vi "VI Linearisierung v2.vi"() -> ()   [LabVIEW 2020, in "Linearisierung v2.lvlib"] (continued)
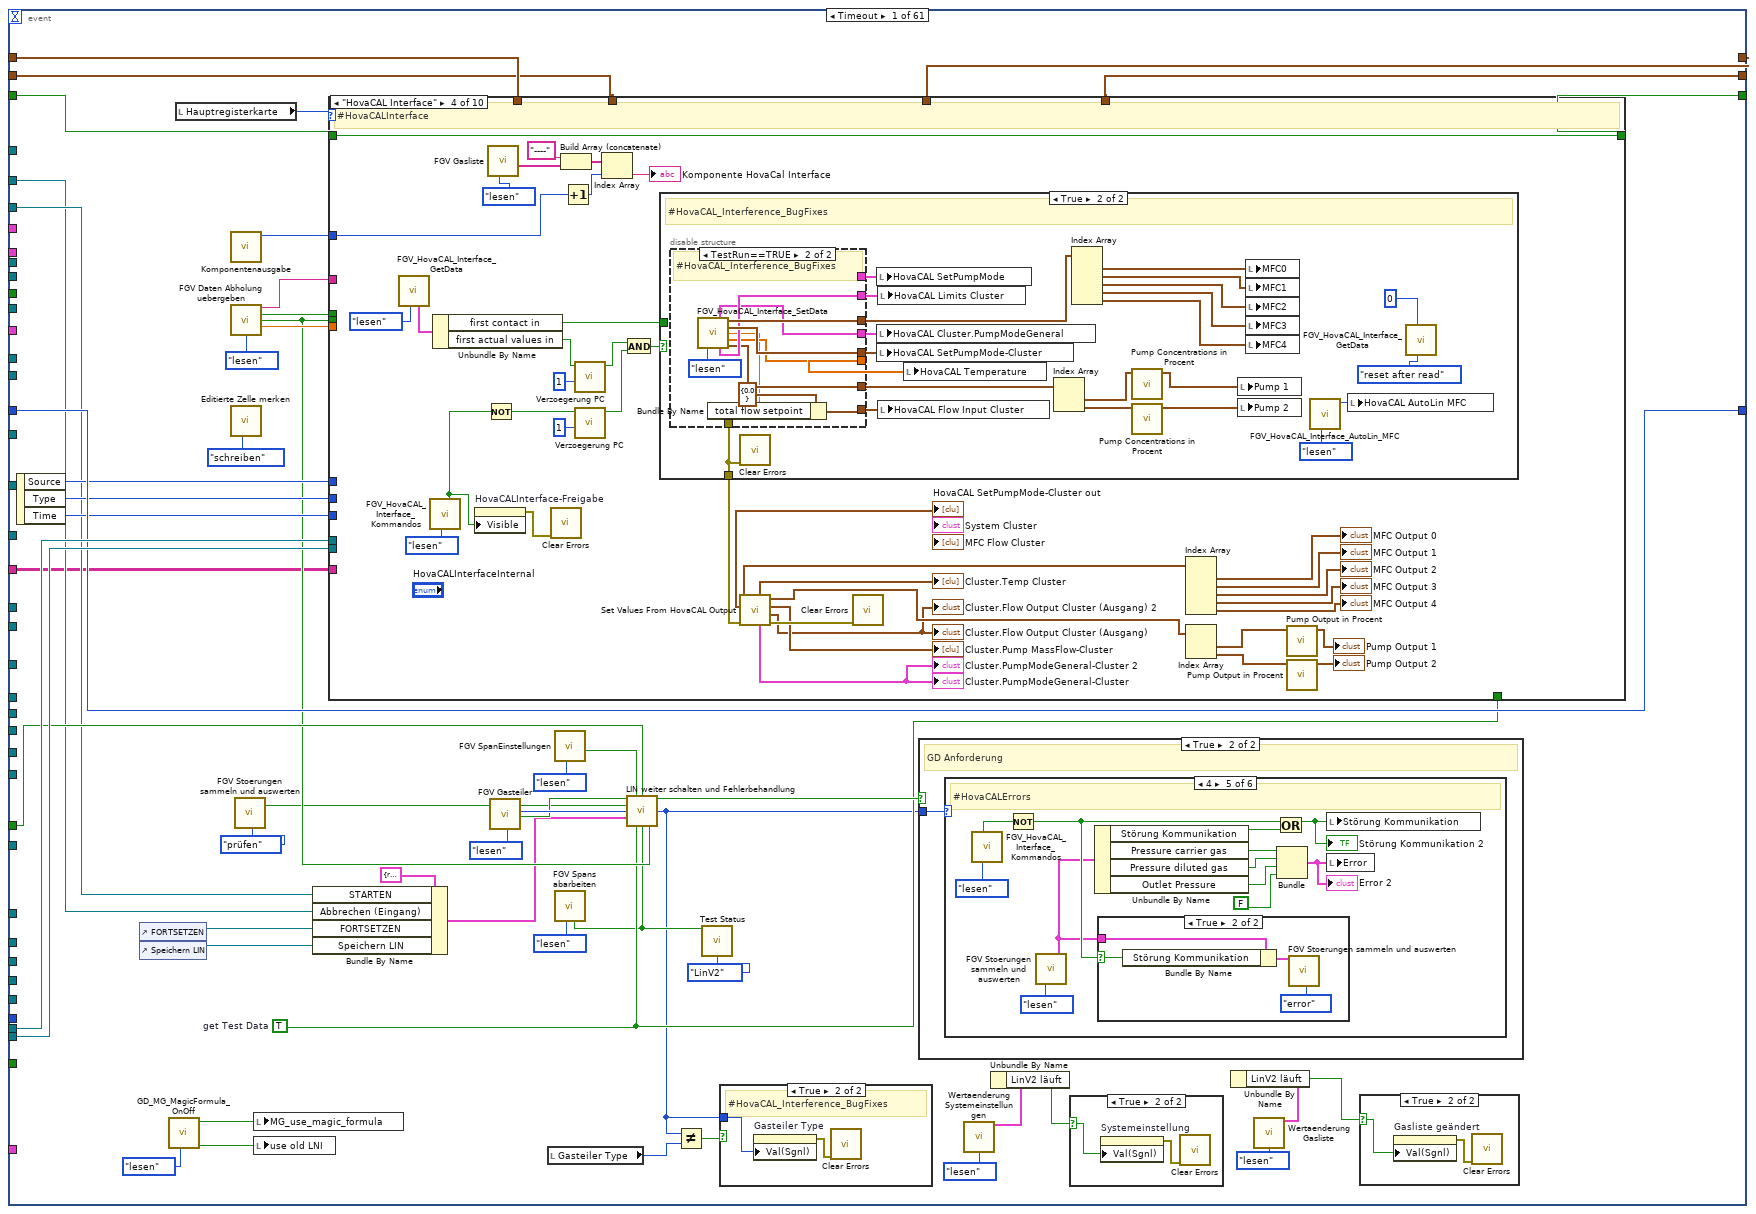
[diagram p2: hidden frame]
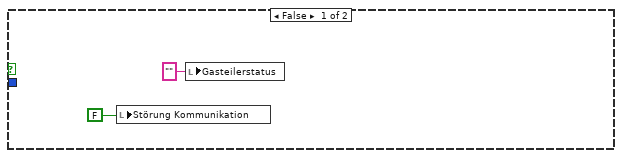
[diagram p6: hidden frame]
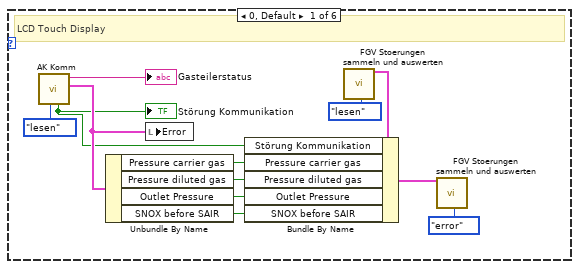
[diagram p7: hidden frame]
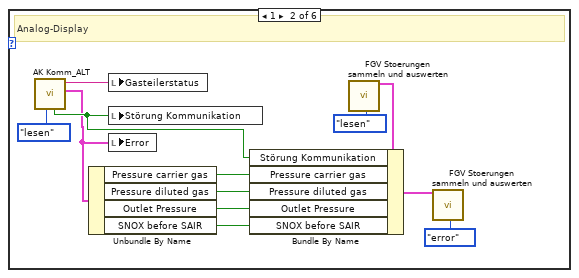
[diagram p8: hidden frame]
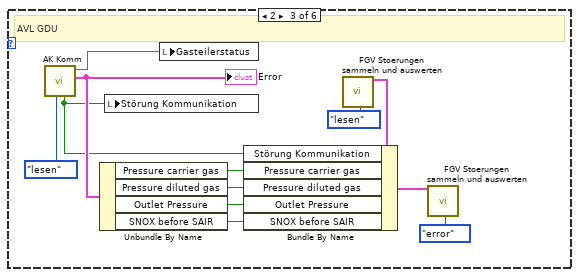
[diagram p9: hidden frame]
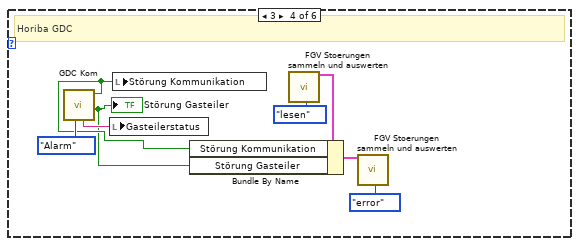
[diagram p10: hidden frame]
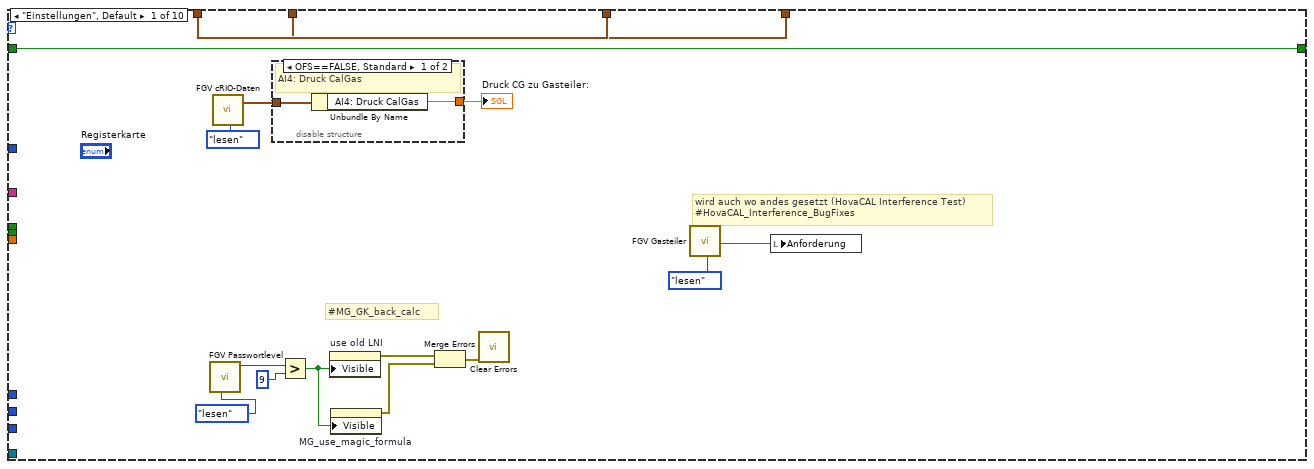
[diagram p13: hidden frame]
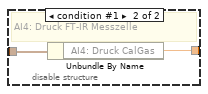
[diagram p14: hidden frame]
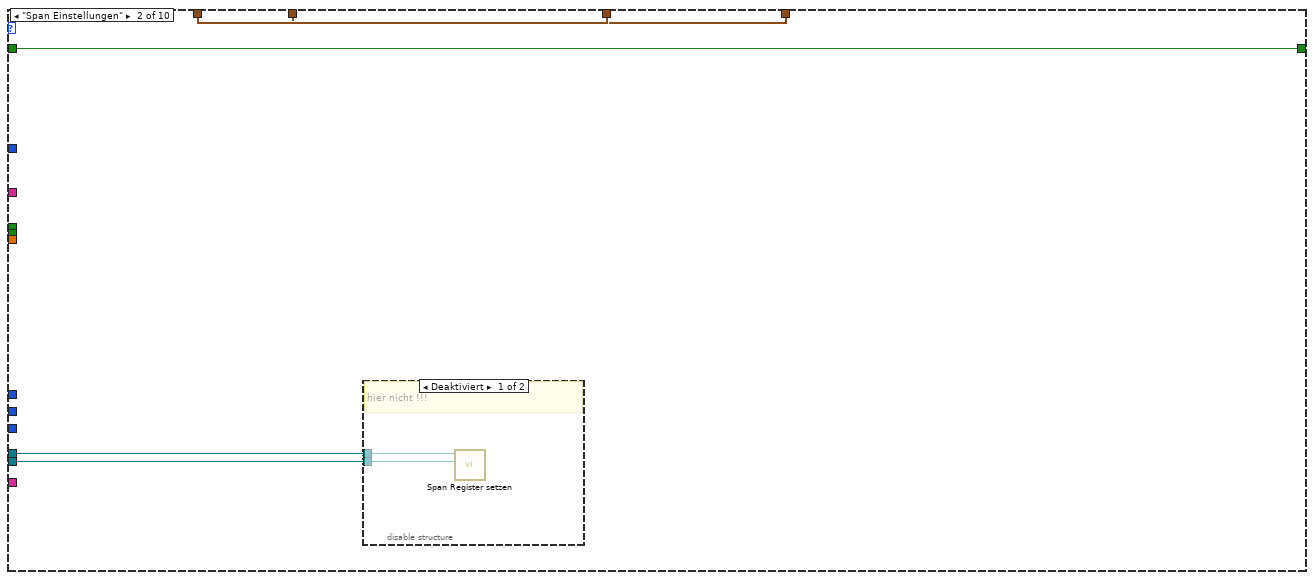
[diagram p15: hidden frame]
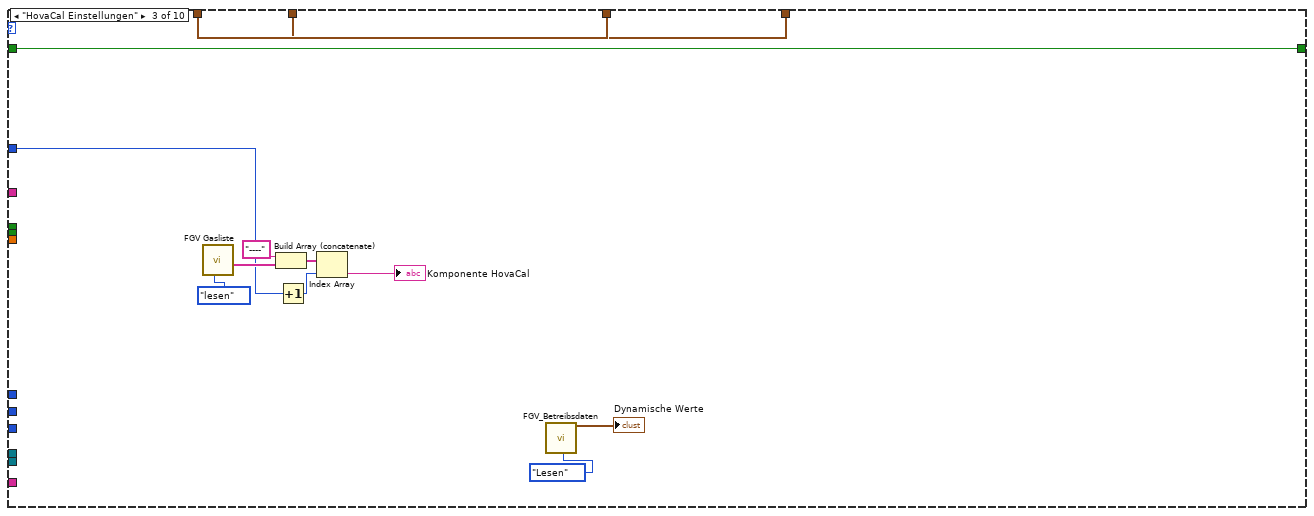
[diagram p17: hidden frame]
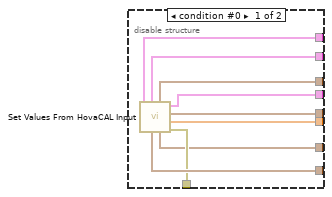
[diagram p19: hidden frame]
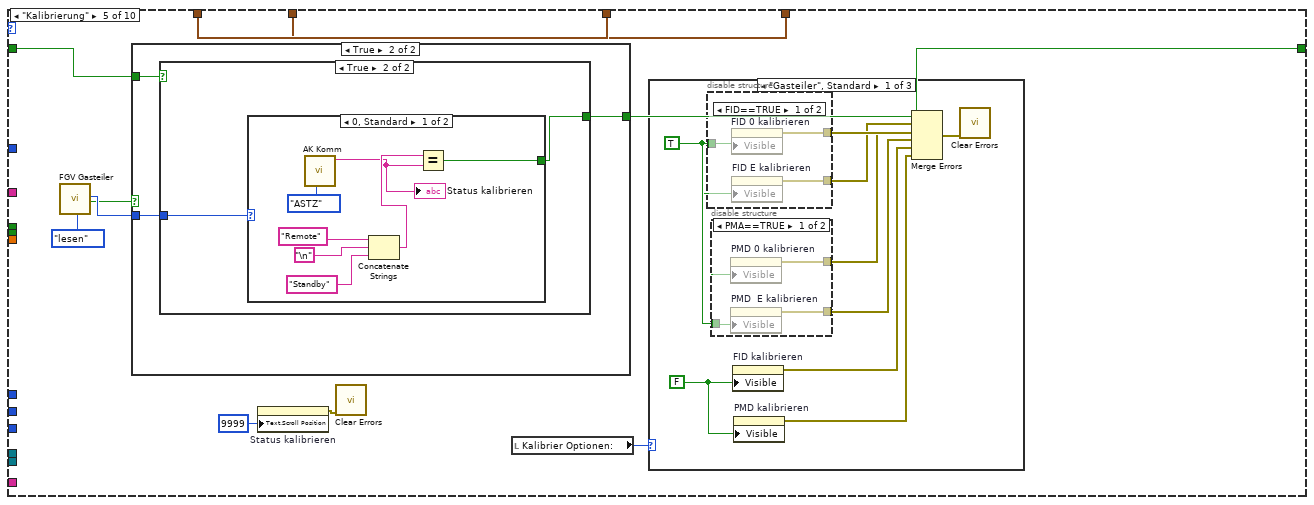
[diagram p20: hidden frame]
                    n2156 = call "FGV_Betreibsdaten.vi"("Enum"=Aktion_FGV_Betriebsdaten."Lesen" ("Aktion")) -> ("Sollwert für Vergleich"=w4010:T64)  [unwired: 11 in, 7 out]
                    n2157 = Bundle By Name(cluster=w4010, "Eingangskonzentration\nKomponente 1"=w4012) -> (w4014:T64)
                    n2158 = call "FGV_Betreibsdaten.vi"("Sollwert schreiben"=w4014, "Enum"=Aktion_FGV_Betriebsdaten."Sollwerte schreiben" ("Aktion")) -> ("Sollwert für Vergleich"=w4011:T64)  [unwired: 10 in, 7 out]
                    n2159 = property on="Daten" class="Cluster (strikt)"("Val(Sgnl)"=w4011) -> (error out=w4013:errorcluster)  [unwired: 2 in, 1 out]
                    n2160 = call <vilib>:"Clear Errors.vi"("error in (no error)"=w4013) -> ()  [unwired: 5 in, 2 out]
                  }
                  frame 2 {
                    n2161 = call "FGV_Betreibsdaten.vi"("Enum"=Aktion_FGV_Betriebsdaten."Lesen" ("Aktion")) -> ("Sollwert für Vergleich"=w4017:T64)  [unwired: 11 in, 7 out]
                    n2162 = Bundle By Name(cluster=w4017, "Eingangskonzentration \nKomponente 2"=w4019) -> (w4021:T64)
                    n2163 = call "FGV_Betreibsdaten.vi"("Sollwert schreiben"=w4021, "Enum"=Aktion_FGV_Betriebsdaten."Sollwerte schreiben" ("Aktion")) -> ("Sollwert für Vergleich"=w4018:T64)  [unwired: 10 in, 7 out]
                    n2164 = property on="Daten" class="Cluster (strikt)"("Val(Sgnl)"=w4018) -> (error out=w4020:errorcluster)  [unwired: 2 in, 1 out]
                    n2165 = call <vilib>:"Clear Errors.vi"("error in (no error)"=w4020) -> ()  [unwired: 5 in, 2 out]
                  }
                }
              }
              frame condition #1 (active) {
                n2166 = call "Expand MFC count 2 max MFC index for Pump index.vi"("AutoLin MFC"=w4025) -> ("Pump"=w4024:bool, "Pump Idx"=w4022:i32)  [unwired: 8 in, 1 out]
                n2167 = call "HovaCAL ppm convert from Component.vi"("Konzentration"=w4028, "Gasnummer"=w4026) -> ("Komponenten Name"=w4023:T48, "Konzentration in ppm"=w4027:dbl)  [unwired: 5 in, 3 out]
                n2168 = case shown="True" w4024 {
                  tunnel: w4027 -> [w4030 _]
                  tunnel: w4025 -> [w4029 _]
                  tunnel: w4023 -> [_ w4032]
                  tunnel: w4022 -> [_ w4031]
                  frame False {
                    # "gas"
                    n2169 = call "HovaCAL_Interface_SetComponentConcentration.vi"("AutoLin MFV Index"=w4029, "Konzentration"=w4030) -> ()  [unwired: 7 in, 3 out]
                  }
                  frame True {
                    # "water/reagent"
                    n2170 = call "HovaCAL_Interface_SetPumpParameter.vi"("Pump Idx"=w4031, "Komponent Name"=w4032) -> ()  [unwired: 9 in, 1 out]
                  }
                }
              }
            }
          }
        }
        n2171 = local write "LIN Polynomkoeffizienten"(w3935) -> ()
        n2172 = Index Array(array=w3899, index=w3900) -> (element=w3898:refnum<vi>)
        n2173 = local write "EPA Ausgabetabelle"(w3939) -> ()
        n2174 = local write "LIN Ausgabetabelle"(w3936) -> ()
        n2175 = local write "EPA Auswertung"(w3937) -> ()
        n2176 = local write "XY-Graph EPA"(w3938) -> ()
        n2177 = property class="Tbl (strikt)"(reference=w3898, "Value"=w3897) -> (error out=w3896:errorcluster)  [unwired: 1 in, 1 out]
        n2178 = local write "Aktiv"(w3940) -> ()
        n2179 = call <vilib>:"Clear Errors.vi"("error in (no error)"=w3896) -> ()  [unwired: 5 in, 2 out]
      }
      event Value Change {
        # "Stufenaufteilung immer nur nach 1. Komponente ?!\nFormel daher auch ...\naus Gaxsliste oder aus \"vereinzeln\" ?"
        # "-> Bearbeiter -> Gasnummer generieren"
        n2180 = event-data() -> ()  [unwired: 1 in, 6 out]
        n2181 = Build Array("Span 1", "Span 2", "Span 3", "Span 4", "Span 5", "Span 6", "Span 7", "Span 8", "Span 9", "Span 10") -> (w4064:T19[])
        n2182 = call "FGV SpanEinstellungen.vi"("Aktion"=Aktion_FGV_SpanEinstellungen."lesen") -> ("SpanInletClusterArray out"=w4062:T19[])  [unwired: 6 in, 4 out]
        n2183 = for {
          tunnel: w4065 -> [w4094] mode=indexing
          tunnel: w4064 -> [w4088] mode=indexing
          tunnel: w4062 -> [w4093] mode=indexing
          tunnel: [w4087] -> w4049 mode=indexing
          n2184 = call "FGV SPAN Verriegelung.vi"("aktion"=Aktion_FGV_SPAN_Verriegelung."lesen") -> ("locked"=w4081:bool)  [unwired: 8 in, 2 out]
          n2185 = Unbundle By Name(w4088) -> ("Konfig Gasflasche"=w4091:T20, "Komponenten"=w4085:T23, "Gasflasche"=w4089:T22)
          n2186 = Unbundle By Name(w4093) -> ("Komponenten"=w4086:T23, "Gasflasche"=w4092:T22)
          n2187 = case shown="False" w4081 {
            tunnel: w4094 -> [w4096 _]
            tunnel: w4091 -> [w4095 _]
            frame False {
              n2188 = call "Konfig Gasflasche aktiv.vi"("Konfig Gasflasche"=w4095, "Referenz Gasflasche"=w4096) -> ("error out"=w4097:errorcluster)  [unwired: 9 in]
              n2189 = call <vilib>:"Clear Errors.vi"("error in (no error)"=w4097) -> ()  [unwired: 5 in, 2 out]
            }
            frame True {
            }
          }
          n2190 = Not Equal?(x=w4089, y=w4092) -> (x != y?=w4090:bool)
          n2191 = Not Equal?(x=w4085, y=w4086) -> (x != y?=w4083:bool)
          n2192 = And(x=w4091, y=w4090) -> (x .and. y?=w4082:T20)
          n2193 = case shown="False" w4083 {
            tunnel: w4089 -> [w4101 _]
            tunnel: w4088 -> [w4100 w4109]
            tunnel: [w4099 w4108] -> w4087
            tunnel: w4086 -> [_ w4110]
            tunnel: w4085 -> [_ w4107]
            tunnel: w4082 -> [w4098 _]
            frame False {
              n2194 = case shown="True" w4098 {
                tunnel: w4101 -> [_ w4105]
                tunnel: w4100 -> [w4102 w4104]
                tunnel: [w4102 w4103] -> w4099
                frame False {
                }
                frame True {
                  n2195 = call "Spaneinstellung befuellen.vi"("Gasflasche"=w4105, "Span 1"=w4104) -> ("Span 1"=w4103:T19)  [unwired: 7 in, 2 out]
                }
              }
            }
            frame True {
              n2196 = call "Komponenten Formeln Finden.vi"("Komponenten Alt"=w4110, "Komponenten (Eingang)"=w4107) -> ("Komponenten (Ausgang)"=w4106:T23)  [unwired: 9 in]
              n2197 = Bundle By Name(cluster=w4109, "Komponenten"=w4106) -> (w4108:T19)
            }
          }
        }
        n2198 = call "get Summenformeln and update.vi"("SpanInletClusterArray in"=w4049) -> ("error out"=w4047:errorcluster, "Summenformeln 1.Komponente"=w4046:T12[], "SpanInletClusterArray out"=w4048:T19[])  [unwired: 7 in, 1 out]
        n2199 = Index Array(array=w4046) -> (element #1=w4045:T12, element #2=w4044:T12, element #3=w4043:T12, element #4=w4042:T12, element #5=w4041:T12, element #6=w4040:T12, element #7=w4039:T12, element #8=w4038:T12, element #9=w4037:T12, element #10=w4036:T12)  [unwired: 10 in]
        n2200 = call "FGV SpanEinstellungen.vi"("Aktion"=Aktion_FGV_SpanEinstellungen."schreiben", "error in (no error)"=w4047, "SpanInletClusterArray in"=w4048) -> ("error out"=w4066:errorcluster, "SpanInletClusterArray out"=w4051:T19[])  [unwired: 4 in, 3 out]
        n2201 = local write "PrüfgasName"(w4045) -> ()
        n2202 = local write "PrüfgasName 2"(w4044) -> ()
        n2203 = local write "PrüfgasName 3"(w4043) -> ()
        n2204 = local write "PrüfgasName 4"(w4042) -> ()
        n2205 = local write "PrüfgasName 5"(w4041) -> ()
        n2206 = local write "PrüfgasName 6"(w4040) -> ()
        n2207 = local write "PrüfgasName 7"(w4039) -> ()
        n2208 = local write "PrüfgasName 8"(w4038) -> ()
        n2209 = local write "PrüfgasName 9"(w4037) -> ()
        n2210 = local write "PrüfgasName 10"(w4036) -> ()
        n2211 = call "FGV SpanEinstellungen.vi"("Aktion"=Aktion_FGV_SpanEinstellungen."speichern", "error in (no error)"=w4066, "SpanInletClusterArray in"=w4051) -> ("automatisch out"=w4035:T20, "SpanInletClusterArray out"=w4050:T19[])  [unwired: 4 in, 3 out]
        n2212 = Index Array(array=w4050) -> (element #1=w4061:T19, element #2=w4060:T19, element #3=w4059:T19, element #4=w4058:T19, element #5=w4057:T19, element #6=w4056:T19, element #7=w4055:T19, element #8=w4054:T19, element #9=w4053:T19, element #10=w4052:T19)  [unwired: 10 in]
        n2213 = local write "Span 1"(w4061) -> ()
        n2214 = local write "Span 2"(w4060) -> ()
        n2215 = local write "Span 3"(w4059) -> ()
        n2216 = local write "Span 4"(w4058) -> ()
        n2217 = local write "Span 5"(w4057) -> ()
        n2218 = local write "Span 6"(w4056) -> ()
        n2219 = local write "Span 7"(w4055) -> ()
        n2220 = local write "Span 8"(w4054) -> ()
        n2221 = local write "Span 9"(w4053) -> ()
        n2222 = local write "Span 10"(w4052) -> ()
        n2223 = call "Bearbeiter_triggern.vi"("automatisch out"=w4035, "Bearbeiter (Eingang)"=w4034) -> ()  [unwired: 10 in]
      }
      event Value Change {
        n2224 = event-data() -> ()  [unwired: 1 in, 1 out]
        n2225 = vi-ref "Gasteiler Korrektur.vi"() -> (w4113:refnum<vi>)
        n2226 = call "VI Pop Up.vi"("VI Referenz"=w4113) -> ()  [unwired: 10 in, 1 out]
      }
      event Value Change {
        n2227 = event-data() -> ()  [unwired: 1 in, 1 out]
        n2228 = case shown="True" "Istwerte löschen" {
          tunnel: [_ w4136] -> w4133
          frame False {
          }
          frame True {
            n2229 = call "Lin Daten aufarbeiten.vi"("Aktionen"=Aktion_Lin_Daten_aufarbeiten."Istwerte löschen") -> ("error out"=w4136:errorcluster)  [unwired: 16 in, 10 out]
          }
        }
        n2230 = case shown="True" "Alles löschen" {
          tunnel: [_ w4138] -> w4132
          frame False {
          }
          frame True {
            n2231 = call "Lin Daten aufarbeiten.vi"("Aktionen"=Aktion_Lin_Daten_aufarbeiten."Tabelle löschen") -> ("error out"=w4138:errorcluster)  [unwired: 16 in, 10 out]
          }
        }
        n2232 = Merge Errors(w4133, w4132) -> (w4124:errorcluster)
        n2233 = call "Komponentenausgabe.vi"() -> ("Gaskomponente"=w4119:T7)  [unwired: 8 in, 3 out]
        n2234 = call "Lin Daten aufarbeiten.vi"("Index (Seite)"=w4119, "error in (no error)"=w4124, "Aktionen"=Aktion_Lin_Daten_aufarbeiten."EPA auswerten") -> ("Index (Seite) out"=w4118:i32, "error out"=w4123:errorcluster)  [unwired: 14 in, 9 out]
        n2235 = call "Lin Daten aufarbeiten.vi"("Index (Seite)"=w4118, "error in (no error)"=w4123, "Polynom-Ordnung"=Auswahl_Polynom_Ordnung."actual", "Aktionen"=Aktion_Lin_Daten_aufarbeiten."Lin auswerten") -> ("Index (Seite) out"=w4117:i32, "error out"=w4122:errorcluster)  [unwired: 13 in, 9 out]
        n2236 = call "Lin Daten aufarbeiten.vi"("Index (Seite)"=w4117, "error in (no error)"=w4122, "Aktionen"=Aktion_Lin_Daten_aufarbeiten."lesen") -> ("Eingabetabelle"=w4130:T54, "error out"=w4131:errorcluster)  [unwired: 14 in, 9 out]
        n2237 = call "AusgabeTabelle zusammenbauen.vi"("error in (no error)"=w4131, "Eingabetabelle"=w4130) -> ("Eingabetabelle behandelt"=w4127:string[][], "Ausgabetabelle"=w4128:T53)  [unwired: 7 in, 1 out]
        n2238 = local write "Ausgabetabelle"(w4128) -> ()
        n2239 = local write "Eingabetabelle"(w4127) -> ()
      }
      event Value Change {
        n2240 = event-data() -> ()  [unwired: 1 in, 1 out]
        n2241 = local read "Gasteiler Type"() -> (w4144:T15)
        n2242 = call "FGV Gasteiler.vi"("Serielle Parameter"="Serielle Parameter", "Aktionen"=Aktionen_FGV_Gasteiler_Daten."Seriellen Param.") -> ("Serielle Parameter"=w4148:T129)  [unwired: 10 in, 7 out]
        n2243 = call "FGV Gasteiler.vi"("Serielle Parameter"=w4148, "Aktionen"=Aktionen_FGV_Gasteiler_Daten."speichern") -> ("Serielle Parameter"=w4141:T129)  [unwired: 10 in, 7 out]
        n2244 = case shown="4" w4144 {
          tunnel: w4141 -> [_ w4150]
          frame 0, Default {
          }
          frame 4 {
            # "#HovaCALInterface"
            n2245 = Unbundle By Name(w4150) -> ("VISA resource name"=w4149:refnum<visa-resource-name>)
            n2246 = call "FGV Gasteiler.vi"("Aktionen"=Aktionen_FGV_Gasteiler_Daten."lesen") -> ("Anforderung"=w4151:bool)  [unwired: 11 in, 7 out]
            n2247 = case shown="True" w4151 {
              tunnel: w4149 -> [w4153 w4159]
              frame False {
                n2248 = disable-structure shown="HovaCALInterface==TRUE, Standard" {
                  disable-tunnel: w4153 -> [w4154 _]
                  frame condition #0 {
                    n2249 = call "FGV_Kommunikation.vi"("Aktion"=Aktion_FGV_Kom."Com ändern", "VISA"=w4154) -> ("error out"=w4155:errorcluster)  [unwired: 5 in, 4 out]
                    n2250 = call <vilib>:"Clear Errors.vi"("error in (no error)"=w4155) -> ()  [unwired: 5 in, 2 out]
                  }
                  frame condition #1 (active) {
                    n2251 = call "FGV_HovaCAL_Interface_Kommandos.vi"("Aktion"=Aktion_FGV_HovaCAL_Interface_Kommandos."on top", "Kommando in"=Aktion_FGV_HovaCAL_Interface_Kommunikation."Com ändern" ("Kommando")) -> ()  [unwired: 3 in, 6 out]
                  }
                }
              }
              frame True {
                n2252 = stacked-sequence {
                  tunnel: w4159 -> [w4160 _ _]
                  frame #0 {
                    n2253 = disable-structure shown="HovaCALInterface==TRUE, Standard" {
                      disable-tunnel: w4160 -> [w4161 _]
                      frame condition #0 {
                        n2254 = call "FGV_Kommunikation.vi"("Aktion"=Aktion_FGV_Kom."Beenden") -> ("error out"=w4165:errorcluster)  [unwired: 6 in, 4 out]
                        n2255 = call "FGV_Kommunikation.vi"("error in"=w4165, "Aktion"=Aktion_FGV_Kom."Com ändern", "VISA"=w4161) -> ("error out"=w4163:errorcluster)  [unwired: 4 in, 4 out]
                        n2256 = call "FGV_Kommunikation.vi"("error in"=w4163, "Aktion"=Aktion_FGV_Kom."Initialisieren") -> ("error out"=w4162:errorcluster)  [unwired: 5 in, 4 out]
                        n2257 = call <vilib>:"Clear Errors.vi"("error in (no error)"=w4162) -> ()  [unwired: 5 in, 2 out]
                      }
                      frame condition #1 (active) {
                        n2258 = call "FGV_HovaCAL_Interface_Kommandos.vi"("Aktion"=Aktion_FGV_HovaCAL_Interface_Kommandos."on top", "Kommando in"=Aktion_FGV_HovaCAL_Interface_Kommunikation."Com ändern" ("Kommando")) -> ("error out"=w4168:errorcluster)  [unwired: 3 in, 5 out]
                        n2259 = disable-structure shown="Deaktiviert" {
                          disable-tunnel: w4168 -> [w4171 _]
                          frame Disabled {
                            n2260 = call "FGV_HovaCAL_Interface_Kommandos.vi"("Aktion"=Aktion_FGV_HovaCAL_Interface_Kommandos."on top", "error in"=w4171, "Kommando in"=Aktion_FGV_HovaCAL_Interface_Kommunikation."Beenden" ("Kommando")) -> ()  [unwired: 2 in, 6 out]
                          }
                          frame Enabled {
                          }
                        }
                      }
                    }
                  }
                  frame #1 {
                    n2261 = disable-structure shown="HovaCALInterface==TRUE, Standard" {
                      frame condition #0 {
                        n2262 = Wait (ms)(milliseconds to wait=u32 2000 ("Zu wartende ms")) -> ()  [unwired: 1 out]
                      }
                      frame condition #1 (active) {
                      }
                    }
                  }
                  frame #2 {
                    n2263 = disable-structure shown="HovaCALInterface==FALSE" {
                      frame condition #0 {
                        n2264 = call "FGV_Kommunikation.vi"("Aktion"=Aktion_FGV_Kom."Gase init") -> ("error out"=w4178:errorcluster, "Gase"=w4176:cluster{string, i32}[][])  [unwired: 6 in, 3 out]
                        n2265 = call "FGV_Betreibsdaten.vi"("Strings und Werte"=w4176, "error in (no error)"=w4178, "Enum"=Aktion_FGV_Betriebsdaten."Gase aendern") -> ("error out"=w4177:errorcluster)  [unwired: 9 in, 7 out]
                        n2266 = call <vilib>:"Clear Errors.vi"("error in (no error)"=w4177) -> ()  [unwired: 5 in, 2 out]
                      }
                      frame condition #1 (active) {
                      }
                    }
                  }
                }
              }
            }
          }
        }
      }
      event "Gasteiler Span Eingänge": Value Change {
        # "#Option10xSpanAuto"
        n2267 = event-data() -> ()  [unwired: 1 in, 1 out]
        n2268 = call "Lin Daten aufarbeiten.vi"("Aktionen"=Aktion_Lin_Daten_aufarbeiten."lesen") -> ("Lin-Polynom"=w4235:T119)  [unwired: 16 in, 10 out]
        n2269 = Bundle By Name(cluster=w4235, "Kalibrator (Gasteiler)"="Gasteiler") -> (w4232:T119)
        n2270 = case shown="4" "Gasteiler Type" {
          selector: "Gasteiler Type" -> [w4285 _ _ _]
          tunnel: "Gasteiler Stufen" -> [w4291 w4300 w4309 _]
          tunnel: [w4291 w4300 w4309 w4322] -> w4228
          tunnel: [FALSE w4299 w4305 w4313] -> w4194
          tunnel: [w4288 w4299 w4307 w4313] -> w4209
          tunnel: [w4288 w4299 w4307 w4313] -> w4208
          tunnel: [w4289 w4298 w4308 TRUE] -> w4207
          tunnel: [w4288 w4299 w4307 w4313] -> w4206
          tunnel: [w4288 w4298 w4307 w4313] -> w4205
          tunnel: [w4288 w4298 w4307 w4313] -> w4204
          tunnel: [w4288 w4299 w4307 w4313] -> w4203
          tunnel: [w4288 w4299 w4307 w4313] -> w4202
          tunnel: [w4288 w4299 w4306 w4313] -> w4201
          tunnel: [w4288 w4299 w4306 w4313] -> w4200
          tunnel: [w4288 w4299 w4306 w4313] -> w4199
          tunnel: [w4288 w4299 w4306 w4313] -> w4198
          tunnel: [w4288 w4299 w4306 w4313] -> w4197
          tunnel: [w4288 w4299 w4305 w4313] -> w4196
          tunnel: [w4288 w4298 w4307 w4313] -> w4195
          tunnel: [FALSE _ TRUE _] -> w4193
          tunnel: w4192 -> [w4277 w4295 w4301 _]
          tunnel: [w4277 w4295 w4301 w4311] -> w4188
          tunnel: w4191 -> [w4286 w4294 w4303 _]
          tunnel: [w4286 w4294 w4303 w4313] -> w4190
          tunnel: "Gasteiler Span Eingänge" -> [w4282 _ w4302 _]
          tunnel: [w4281 0 ("y") w4302 0 ("y")] -> w4186
          tunnel: [w4278 T66."Disabled and Grayed Out" ("Deaktiviert") w4301 w4311] -> w4181
          frame 0..2, Default {
            w4284 = T15 0 items=["LNI", "Analog-Display", "AVL GDU", "Horiba GDC", "HovaCal", "Horiba SGD 710C"] ("x")
            w4288 = TRUE
            # "LCD-Touch Display - Analog Display - AVL GDU"
            n2271 = Equal?(x=w4284, y=w4285) -> (x = y?=w4283:bool)
            n2272 = Select(t=w4277, s=w4283, f=T66."Disabled and Grayed Out" ("Deaktiviert")) -> (s? t:f=w4278:T66)
            n2273 = Not(x=w4288) -> (.not. x?=w4289:bool)
            n2274 = Select(t=w4282, s=w4283, f=u16 0) -> (s? t:f=w4281:u16)
          }
          frame 3 {
            w4296 = FALSE ("Boolesch")
            w4299 = TRUE
            w4298 = FALSE
            # "Horiba GDC"
            n2275 = Boolean To (0,1)(Boolean=w4296) -> (0, 1=w4297:i16)
            n2276 = local write "TCP Verbindung aktiv"(w4296) -> ()
            n2277 = local write "Registerkarte"(w4297) -> ()
          }
          frame 4 {
            w4305 = FALSE
            w4307 = TRUE
            # "Hovacal"
            n2278 = disable-structure shown="HovaCALInterface==TRUE, Standard" {
              disable-tunnel: [TRUE _] -> w4306
              frame condition #0 (active) {
              }
              frame condition #1 {
              }
            }
            n2279 = Not(x=w4307) -> (.not. x?=w4308:bool)
          }
          frame 5 {
            w4311 = T66."Disabled and Grayed Out" ("Deaktiviert")
            w4313 = FALSE
            w4322 = T16 10 items=["10"=10, "16"=16, "32"=32, "64"=64, "128"=128, "256"=256, "500"=500] ("Gasteiler Stufen")
            # "Horiba SGD 710C (manuell)"
            n2280 = local write "Gasteiler Stufen"(w4322) -> ()
            n2281 = call "FGV SpanEinstellungen.vi"("Aktion"=Aktion_FGV_SpanEinstellungen."lesen") -> ("SpanInletClusterArray out"=w4319:T19[])  [unwired: 6 in, 4 out]
            n2282 = To Single Precision Float(number=w4322) -> (single precision float=w4318:sgl)
            n2283 = for {
              tunnel: w4319 -> [w4325] mode=indexing
              tunnel: w4318 -> [w4324]
              tunnel: [w4323] -> w4316 mode=indexing
              n2284 = Bundle By Name(cluster=w4325, "Anzahl Stufen"=w4324) -> (w4323:T19)
            }
            n2285 = call "FGV SpanEinstellungen.vi"("Aktion"=Aktion_FGV_SpanEinstellungen."schreiben", "SpanInletClusterArray in"=w4316) -> ("error out"=w4314:errorcluster)  [unwired: 5 in, 4 out]
            n2286 = call "FGV SpanEinstellungen.vi"("Aktion"=Aktion_FGV_SpanEinstellungen."speichern", "error in (no error)"=w4314) -> ()  [unwired: 5 in, 5 out]
          }
        }
        n2287 = call "Lin Daten aufarbeiten.vi"("Lin-Polynom"=w4232, "Aktionen"=Aktion_Lin_Daten_aufarbeiten."Protkolldaten") -> ()  [unwired: 15 in, 11 out]
        n2288 = case shown="False" w4193 {
          frame True {
            n2289 = control-ref of="Hauptregisterkarte"() -> (w4246:refnum<vi>)
            n2290 = property class="RKElem (strikt)"(reference=w4246) -> (error out=w4249:errorcluster, "Pages"=w4247:refnum<vi>[])  [unwired: 1 in, 1 out]
            n2291 = To Word Integer(number=T8."HovaCal Einstellungen" ("Hauptregisterkarte")) -> (16bit integer=w4245:i16)
            n2292 = Index Array(array=w4247, index #1=w4245, index #2=T8."HovaCAL Interface" ("Hauptregisterkarte")) -> (element #1=w4248:refnum<vi>, element #2=w4250:refnum<vi>)
            n2293 = disable-structure shown="HovaCALInterface==TRUE, Standard" {
              disable-tunnel: w4248 -> [w4257 w4264]
              disable-tunnel: w4249 -> [w4252 w4259]
              disable-tunnel: w4250 -> [w4253 w4260]
              frame condition #0 (active) {
                n2294 = property class="Seite"(reference=w4257, error in=w4252, "PageVis"=FALSE ("Seite sichtbar")) -> (error out=w4255:errorcluster)  [unwired: 1 out]
                n2295 = property class="Seite"(reference=w4253, error in=w4252, "PageVis"=TRUE ("Seite sichtbar")) -> (error out=w4254:errorcluster)  [unwired: 1 out]
                n2296 = call <vilib>:"Clear Errors.vi"("error in (no error)"=w4255) -> ()  [unwired: 5 in, 2 out]
                n2297 = call <vilib>:"Clear Errors.vi"("error in (no error)"=w4254) -> ()  [unwired: 5 in, 2 out]
              }
              frame condition #1 {
                n2298 = property class="Seite"(reference=w4264, error in=w4259, "PageVis"=TRUE ("Seite sichtbar")) -> (error out=w4262:errorcluster)  [unwired: 1 out]
                n2299 = property class="Seite"(reference=w4260, error in=w4259, "PageVis"=FALSE ("Seite sichtbar")) -> (error out=w4261:errorcluster)  [unwired: 1 out]
                n2300 = call <vilib>:"Clear Errors.vi"("error in (no error)"=w4262) -> ()  [unwired: 5 in, 2 out]
                n2301 = call <vilib>:"Clear Errors.vi"("error in (no error)"=w4261) -> ()  [unwired: 5 in, 2 out]
              }
            }
          }
          frame False {
            n2302 = control-ref of="Hauptregisterkarte"() -> (w4272:refnum<vi>)
            n2303 = property class="RKElem (strikt)"(reference=w4272) -> (error out=w4275:errorcluster, "Pages"=w4273:refnum<vi>[])  [unwired: 1 in, 1 out]
            n2304 = To Word Integer(number=T8."HovaCal Einstellungen" ("Hauptregisterkarte")) -> (16bit integer=w4271:i16)
            n2305 = Index Array(array=w4273, index #1=w4271, index #2=T8."HovaCAL Interface" ("Hauptregisterkarte")) -> (element #1=w4274:refnum<vi>, element #2=w4276:refnum<vi>)
            n2306 = property class="Seite"(reference=w4274, error in=w4275, "PageVis"=FALSE ("Seite sichtbar")) -> (error out=w4269:errorcluster)  [unwired: 1 out]
            n2307 = property class="Seite"(reference=w4276, error in=w4275, "PageVis"=FALSE ("Seite sichtbar")) -> (error out=w4268:errorcluster)  [unwired: 1 out]
            n2308 = call <vilib>:"Clear Errors.vi"("error in (no error)"=w4269) -> ()  [unwired: 5 in, 2 out]
            n2309 = call <vilib>:"Clear Errors.vi"("error in (no error)"=w4268) -> ()  [unwired: 5 in, 2 out]
          }
        }
        n2310 = call "FGV Gasteiler.vi"("Aktionen"=Aktionen_FGV_Gasteiler_Daten."lesen") -> ("Gasteiler Daten"=w4241:T118)  [unwired: 11 in, 7 out]
        n2311 = Bundle By Name(cluster=w4241, "Gasteiler"="Gasteiler", "Gasteiler Stufen"=w4228, "Gasteiler Type"="Gasteiler Type", "Gasteiler Span Eingänge"=w4186) -> (w4242:T118)
        n2312 = property on="Störung Gasteiler" class="Bool. (strikt)"("Visible"=w4196) -> (error out=w4225:errorcluster)  [unwired: 2 in, 1 out]
        n2313 = property on="Horiba GDC" class="Bool."("Visible"=w4194) -> (error out=w4226:errorcluster)  [unwired: 2 in, 1 out]
        n2314 = property on="STARTEN" class="Bool. (strikt)"("Visible"=w4208) -> (error out=w4210:errorcluster)  [unwired: 2 in, 1 out]
        n2315 = property on="parity" class="Ring (strikt)"("Visible"=w4199) -> (error out=w4220:errorcluster)  [unwired: 2 in, 1 out]
        n2316 = property on="stop bits" class="Ring (strikt)"("Visible"=w4200) -> (error out=w4221:errorcluster)  [unwired: 2 in, 1 out]
        n2317 = property on="Baud Rate" class="Ring (strikt)"("Visible"=w4197) -> (error out=w4222:errorcluster)  [unwired: 2 in, 1 out]
        n2318 = property on="flow control" class="Ring (strikt)"("Visible"=w4201) -> (error out=w4223:errorcluster)  [unwired: 2 in, 1 out]
        n2319 = property on="data bits" class="Ring (strikt)"("Visible"=w4198) -> (error out=w4224:errorcluster)  [unwired: 2 in, 1 out]
        n2320 = property on="Gasteilerkorrektur" class="Bool."("Visible"=w4207) -> (error out=w4212:errorcluster)  [unwired: 2 in, 1 out]
        n2321 = property on="Registerkarte" class="RKElem (strikt)"("Visible"=w4202) -> (error out=w4218:errorcluster)  [unwired: 2 in, 1 out]
        n2322 = property on="Error" class="Cluster (strikt)"("Visible"=w4195) -> (error out=w4217:errorcluster)  [unwired: 2 in, 1 out]
        n2323 = property on="Störung Kommunikation" class="Bool. (strikt)"("Visible"=w4203) -> (error out=w4216:errorcluster)  [unwired: 2 in, 1 out]
        n2324 = property on="TCP Verbindung aktiv" class="Bool. (strikt)"("Visible"=w4204) -> (error out=w4215:errorcluster)  [unwired: 2 in, 1 out]
        n2325 = property on="Error" class="Cluster (strikt)"("Visible"=w4205) -> (error out=w4214:errorcluster)  [unwired: 2 in, 1 out]
        n2326 = property on="automatisch" class="Bool. (strikt)"("Val(Sgnl)"=w4190, "DisabledEnum"=w4188) -> (error out=w4189:errorcluster)  [unwired: 2 in, 1 out]
        n2327 = property on="Anforderung" class="Bool. (strikt)"("Visible"=w4206) -> (error out=w4213:errorcluster)  [unwired: 2 in, 1 out]
        n2328 = property on="ABBRECHEN" class="Bool."("Visible"=w4209) -> (error out=w4211:errorcluster)  [unwired: 2 in, 1 out]
        n2329 = property on="Gasteiler Span Eingänge" class="Ring (strikt)"("Value"=w4186, "DisabledEnum"=w4181) -> (error out=w4185:errorcluster)  [unwired: 2 in, 1 out]
        n2330 = call "FGV Gasteiler.vi"("Gasteiler Daten"=w4242, "Aktionen"=Aktionen_FGV_Gasteiler_Daten."Gasteiler Daten") -> ("Serielle Parameter"=w4240:T129)  [unwired: 10 in, 7 out]
        n2331 = call "Span Register setzen.vi"("error in (no error)"=w4185, "GD Span Eingänge"=w4183, "automatisch Boolesch (Eingang)"=w4184) -> ("error out"=w4182:errorcluster)  [unwired: 2 in, 6 out]
        n2332 = call "FGV Gasteiler.vi"("Serielle Parameter"=w4240, "Aktionen"=Aktionen_FGV_Gasteiler_Daten."speichern") -> ()  [unwired: 10 in, 8 out]
        n2333 = Merge Errors(w4182, w4189, w4212, w4218, w4217, w4216, w4215, w4214, w4213, w4211, w4210, w4220, w4221, w4222, w4223, w4224, w4225, w4226) -> (w4219:errorcluster)
        n2334 = call <vilib>:"Clear Errors.vi"("error in (no error)"=w4219) -> ()  [unwired: 5 in, 2 out]
      }
      event Value Change {
        w4326 = FALSE
        # "#RickQuickTest_Features"
        # "#PDF_manu_MG"
        n2335 = event-data() -> ()  [unwired: 1 in, 6 out]
        n2336 = call "FGV SpanEinstellungen.vi"("Aktion"=Aktion_FGV_SpanEinstellungen."automatisch", "automatisch in"="automatisch") -> ("error out"=w4350:errorcluster, "SpanInletClusterArray out"=w4351:T19[], "Punkte umkehren und PDF Optionen Cluster"=w4346:T109)  [unwired: 5 in, 2 out]
        n2337 = Unbundle By Name(w4346) -> ("PDF Optionen"=w4345:T108)
        n2338 = Select(t=w4326, s="PDF single pages Span", f=T1 FALSE ("t")) -> (s? t:f=w4333:T1)
        n2339 = Bundle By Name(cluster=w4345, "PDF Einzelseiten Komponenten"="PDF single pages Components", "PDF Einzelseiten Span"="PDF single pages Span", "PDF Deckblatt"="PDF Deckblatt", "PDF öffnen"="PDF öffnen", "Graphik für Messwerte"=w4333) -> (w4337:T108)
        n2340 = case shown="False" "automatisch" {
          tunnel: w4351 -> [w4365 _]
          tunnel: w4350 -> [w4362 w4371]
          tunnel: [w4361 w4371] -> w4342
          tunnel: w4337 -> [w4359 w4370]
          tunnel: [w4358 w4370] -> w4336
          tunnel: [w4357 w4369] -> w4335
          tunnel: [w4357 w4369] -> w4334
          frame False {
            w4357 = T66."Disabled and Grayed Out" ("Deaktiviert")
            w4360 = TRUE ("PDF Einzelseiten Span")
            n2341 = Index Array(array=w4365) -> (element=w4368:T19)  [unwired: 1 in]
            n2342 = Bundle By Name(cluster=w4368, "Span Inlet Active"=T20 TRUE) -> (w4364:T19)
            n2343 = Bundle By Name(cluster=w4359, "PDF Einzelseiten Span"=w4360) -> (w4358:T108)
            n2344 = local write "PDF single pages Span"(w4360) -> ()
            n2345 = Replace Array Subset(array=w4365, new element=w4364) -> (w4363:T19[])  [unwired: 1 in]
            n2346 = call "FGV SpanEinstellungen.vi"("Aktion"=Aktion_FGV_SpanEinstellungen."schreiben", "error in (no error)"=w4362, "SpanInletClusterArray in"=w4363) -> ("error out"=w4361:errorcluster)  [unwired: 4 in, 4 out]
          }
          frame True {
            w4369 = T66."Enabled" ("Deaktiviert")
          }
        }
        n2347 = Select(t=T66."Enabled", s="PDF single pages Span", f=T66."Disabled and Grayed Out" ("Deaktiviert")) -> (s? t:f=w4330:T66)
        n2348 = property on="PDF single pages Span" class="Bool. (strikt)"("DisabledEnum"=w4335) -> ()  [unwired: 2 in, 2 out]
        n2349 = property on="Pfad Auto Lin" class="Pfad (strikt)"("DisabledEnum"=w4334) -> ()  [unwired: 2 in, 2 out]
        n2350 = call "FGV SpanEinstellungen.vi"("Aktion"=Aktion_FGV_SpanEinstellungen."PDF Params", "PDF Optionen"=w4336, "error in (no error)"=w4342) -> ("error out"=w4343:errorcluster)  [unwired: 4 in, 4 out]
        n2351 = property on="Graphik für Messwerte" class="Bool. (strikt)"("Value"=w4326, "DisabledEnum"=w4330) -> (error out=w4332:errorcluster)  [unwired: 2 in, 1 out]
        n2352 = call "FGV SpanEinstellungen.vi"("Aktion"=Aktion_FGV_SpanEinstellungen."speichern", "error in (no error)"=w4343) -> ("error out"=w4352:errorcluster)  [unwired: 5 in, 4 out]
        n2353 = call <vilib>:"Clear Errors.vi"("error in (no error)"=w4332) -> ()  [unwired: 5 in, 2 out]
        n2354 = call "Span Register setzen.vi"("error in (no error)"=w4352, "GD Span Eingänge"=w4347, "automatisch Boolesch (Eingang)"=w4348) -> ()  [unwired: 2 in, 7 out]
      }
      event Value Change {
        n2355 = event-data() -> ()  [unwired: 1 in, 1 out]
        n2356 = flat-sequence {
          frame #0 {
            n2357 = vi-ref "GDC Manuell.vi"() -> (w4375:refnum<vi>)
            n2358 = call "VI Pop Up.vi"("VI Referenz"=w4375) -> ()  [unwired: 10 in, 1 out]
          }
        }
      }
    }
  }
